vi "Browser_for_resources.vi"() -> ()   [LabVIEW 2015]
uses:
  Type Definitions/Data.ctl
  <vilib>/nisyscfg/Close (System).vi
  <vilib>/nisyscfg/nisyscfg.lvlib
panel:
  in  "Tab Control":enum32{"DAQmx", "SERIAL", "GPIB"}(tab)
  out "DAQ devices":bool caption="DAQ devices > 8"
  in  "List DAQ Rsrcs":bool
  out "ProdName":string[](array[string])
  out "DevName":string[](array[string])
  out "DAQ Mess":string caption="Messages"
  in  "Rename DAQ Rsrcs":bool
  in  "DevSerialNum":string
  out "Changed?":bool
  in  "New DevName":string
  out "DevSerialNum":string[](array[string])
  out "SER Mess":string caption="Messages"
  out "COM ports":string[](array[string])
  out "Serial I/F name":string[](array[string]) caption="Interface Instrument Name (RS232)"
  out "Serial Inst ID":string[](array[string]) caption="Instrument ID (RS232)"
  out "Serial List":string[](array[string]) caption="VISA Resource Name (RS232)"
  in  "List SERIAL Rsrcs":bool
  out "SERports >12":bool caption="SERIAL ports > 8"
  out "VISA List":string[](array[string]) caption="VISA Resources list"
  out "GPIB ports >12":bool caption="GPIB ports >8"
  out "Pr. Address":u16[](array[numeric])
  out "GPIB Inst ID":string[](array[string]) caption="Instrument ID (GPIB)"
  out "GPIB I/F name":string[](array[string]) caption="Interface Instrument Name (GPIB)"
  out "GPIB List":string[](array[string]) caption="VISA Resource Name (GPIB)"
  in  "List GPIB Rsrcs":bool
  out "GPIB Mess":string caption="Messages"
  out "VISA List 2":string[](array[string]) caption="VISA Resources list"
  in  "Exit":bool
  # "Browser for Resources (DAQmx, GPIB (INSTR) & SERIAL(INSTR)"
  # "Change DevName"
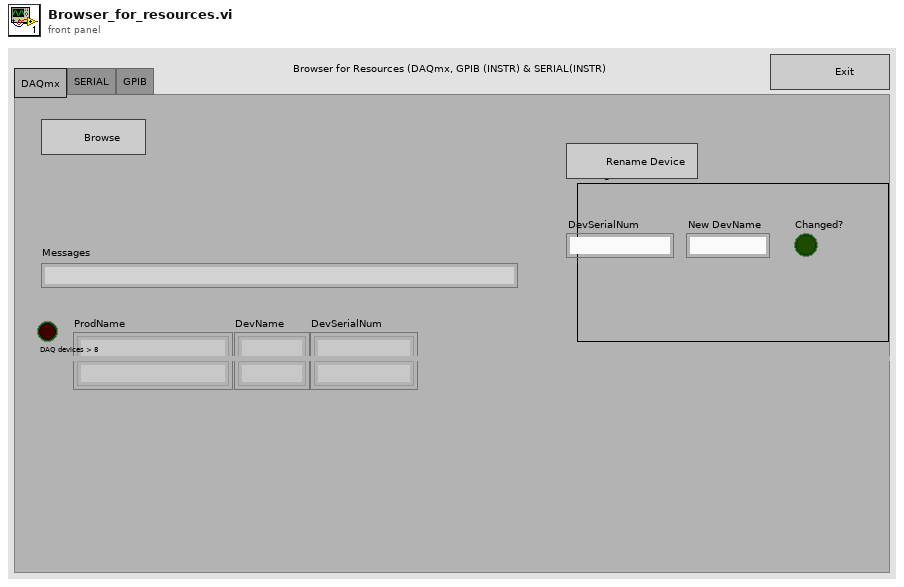
[diagram p1: front panel]
types:
  T1 = typedef "Data.ctl" = cluster{"Resources out":refnum<k20>[], "ProdName":string[], "DAQ Session":refnum<k21>, "DevName":string[], "DAQ Mess":string, "Changed?":bool, "VISA Rsrc":string[], "SERIAL Rsrc":string[], "SERIAL Inst ID":string[], "COM ports":string[], "SERIAL I/F name":string[], "SERIAL rows":u32, "SERIAL Mess":string, "GPIB Rsrc":string[], "GPIB Inst ID":string[], "Pr. Address":u16[], "GPIB I/F name":string[], "GPIB Mess":string, "GPIB rows":u32, "SerialNum":string[]}
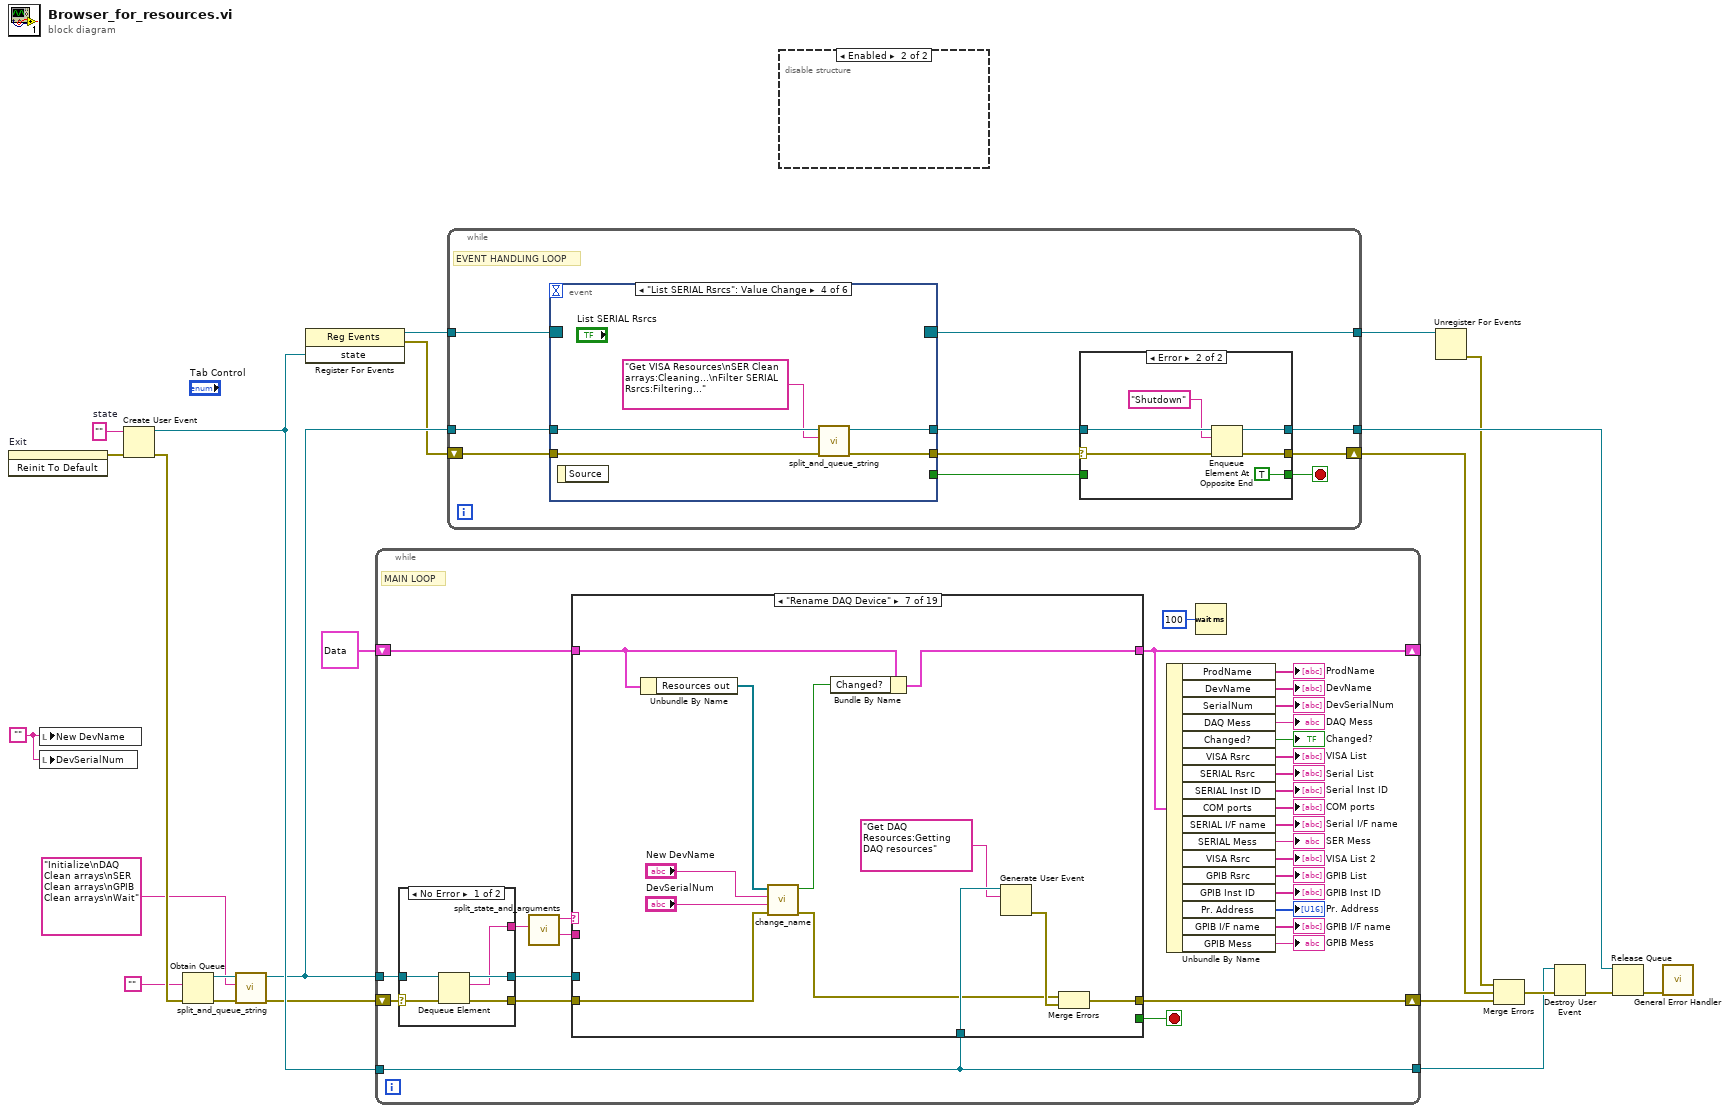
[diagram p0: block diagram]
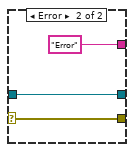
[diagram p3: hidden frame]
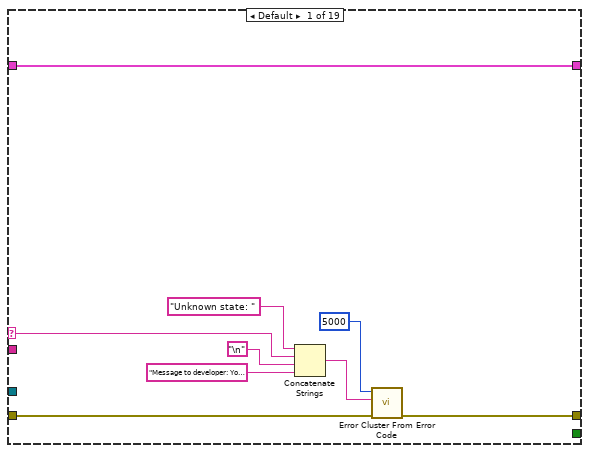
[diagram p4: hidden frame]
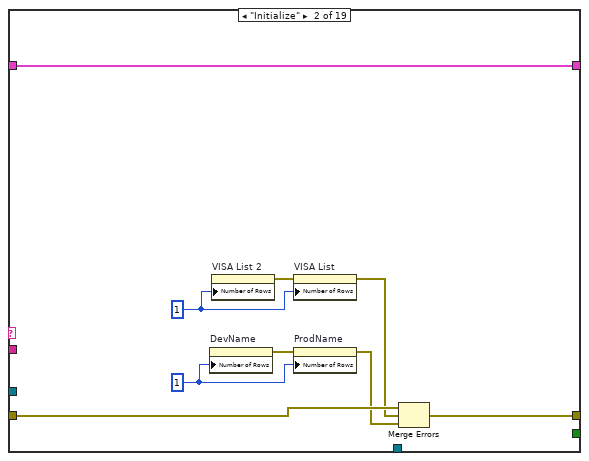
[diagram p5: hidden frame]
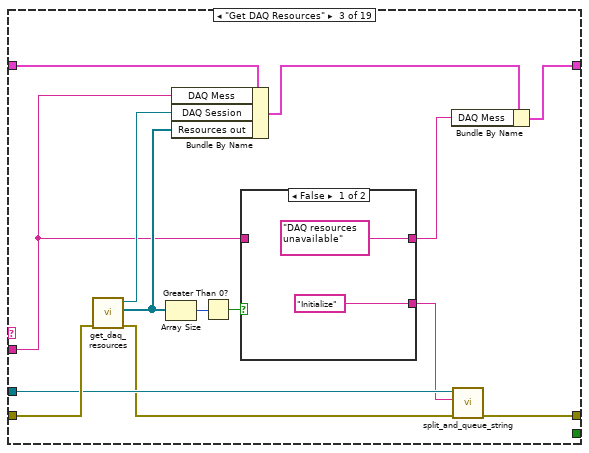
[diagram p6: hidden frame]
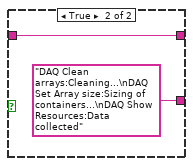
[diagram p7: hidden frame]
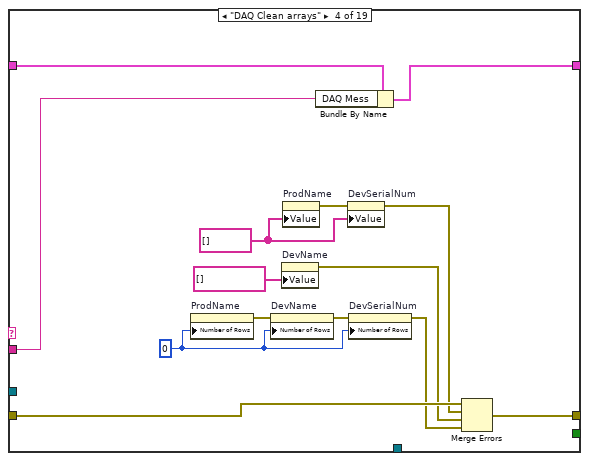
[diagram p8: hidden frame]
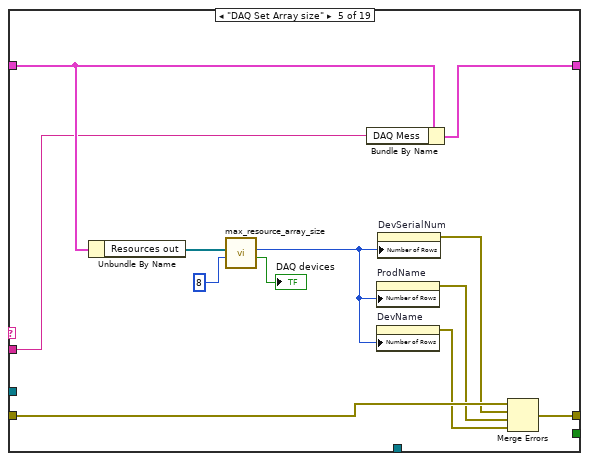
[diagram p9: hidden frame]
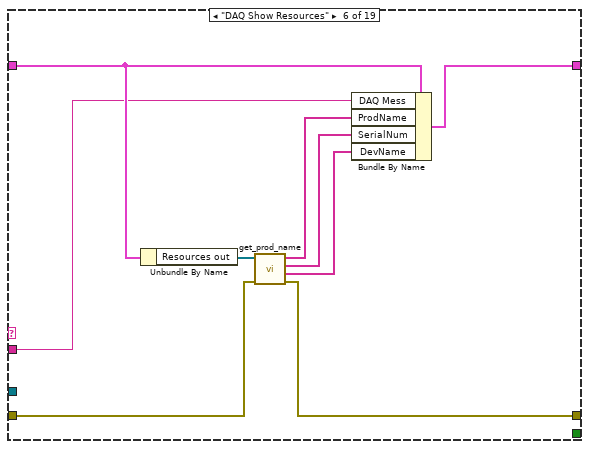
[diagram p10: hidden frame]
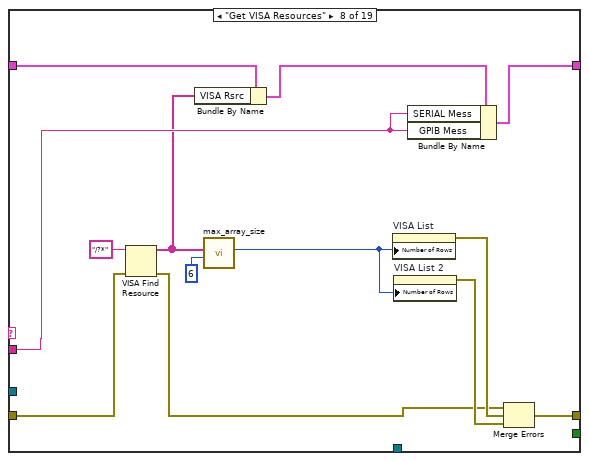
[diagram p11: hidden frame]
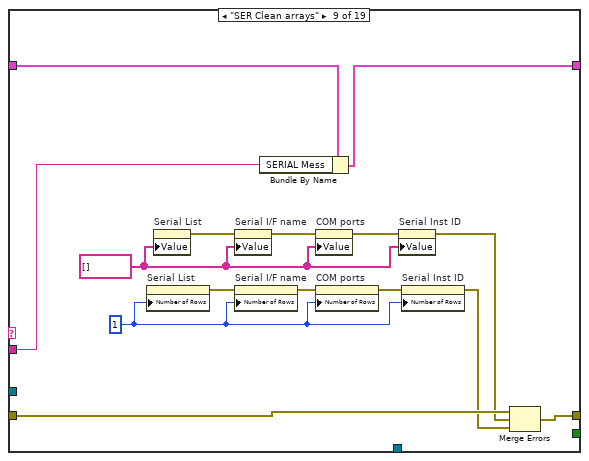
[diagram p12: hidden frame]
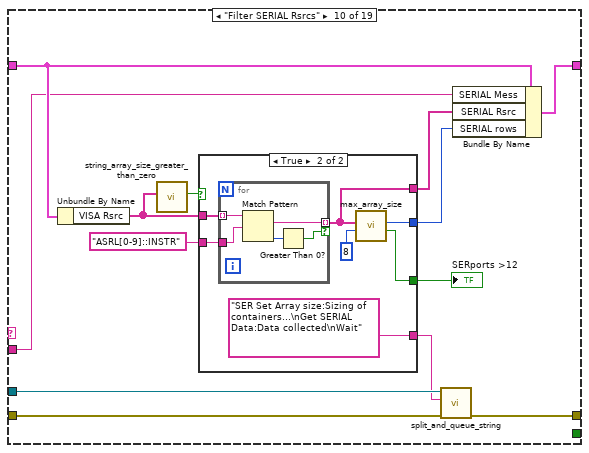
[diagram p13: hidden frame]
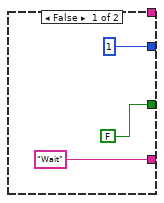
[diagram p14: hidden frame]
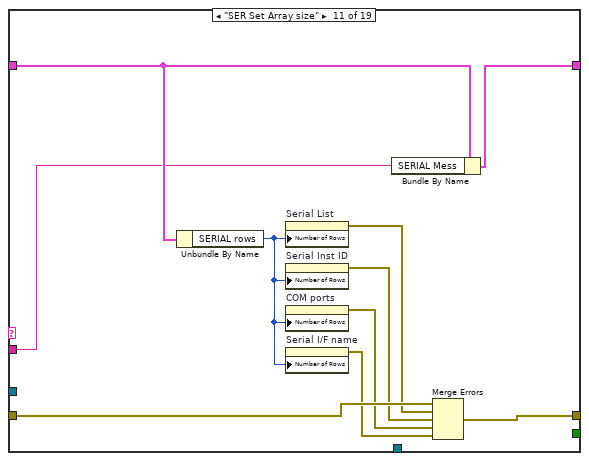
[diagram p15: hidden frame]
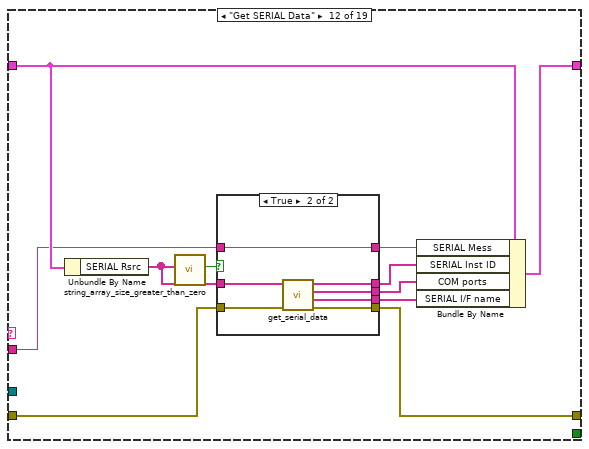
[diagram p16: hidden frame]
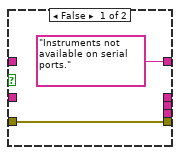
[diagram p17: hidden frame]
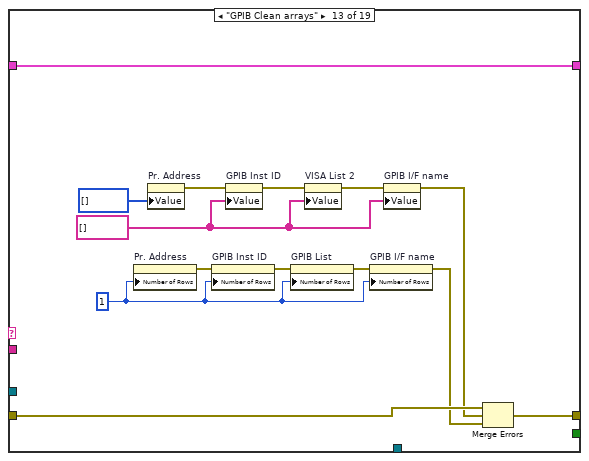
[diagram p18: hidden frame]
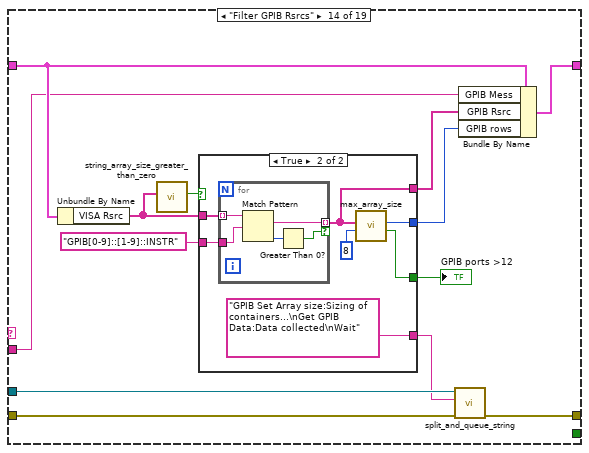
[diagram p19: hidden frame]
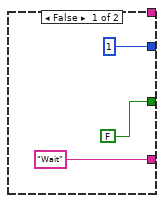
[diagram p20: hidden frame]
diagram:
  w1 = ""
  w13 = ""  # state
  n1 = invoke on="Exit" class="Bool (strict)" method="Reinit To Default"() -> (error out=w4:errorcluster)  [unwired: 3 in, 2 out]
  n2 = local write "New DevName"(w1) -> ()
  n3 = local write "DevSerialNum"(w1) -> ()
  n4 = Create User Event(user event datatype=w13, error in=w4) -> (user event=w23:refnum<user-event>, error out=w5:errorcluster)
  n5 = Obtain Queue(element data type="", error in (no error)=w5) -> (queue out=w21:refnum<queue>, error out=w22:errorcluster)  [unwired: 3 in, 1 out]
  n6 = call "split_and_queue_string.vi"("error in (no error)"=w22, "program string"="Initialize\nDAQ Clean arrays\nSER Clean arrays\nGPIB Clean arrays\nWait", "queue in"=w21) -> ("error out"=w6:errorcluster, "queue out"=w16:refnum<queue>)  [unwired: 7 in]
  n7 = register-events(w23) -> (reference out=w14:refnum<event-registration>, error out=w7:errorcluster)  [unwired: 2 in]
  n8 = while {
    shift-right: [w51] -> w20
    shift-left: w6 -> [w53]
    tunnel: w16 -> [w49]
    shift-right: [w43] -> _
    shift-left: T1 {"Resources out"=[], "ProdName"=[], "DAQ Session"="", "DevName"=[], "DAQ Mess"="", "Changed?"=FALSE, "VISA Rsrc"=[], "SERIAL Rsrc"=[], "SERIAL Inst ID"=[], "COM ports"=[], "SERIAL I/F name"=[], "SERIAL rows"=0, "SERIAL Mess"="", "GPIB Rsrc"=[], "GPIB Inst ID"=[], "Pr. Address"=[], "GPIB I/F name"=[], "GPIB Mess"="", "GPIB rows"=0, "SerialNum"=[]} -> [w44]
    tunnel: w23 -> [w24]
    tunnel: [w24] -> w8
    stop <- w50 stop-if-true
    # "MAIN LOOP"
    n9 = case shown="No Error" w53 {
      selector: w53 -> [w58 w61]
      tunnel: [w55 w61] -> w52
      tunnel: w49 -> [w57 w59]
      tunnel: [w54 "Error"] -> w47
      tunnel: [w56 w59] -> w48
      frame No Error {
        n10 = Dequeue Element(queue=w57, error in (no error)=w58) -> (queue out=w56:refnum<queue>, element=w54:string, error out=w55:errorcluster)  [unwired: 1 in, 1 out]
      }
      frame Error {
      }
    }
    n11 = call "split_state_and_arguments.vi"("String"=w47) -> ("Arguments"=w45:string, "State"=w46:string)  [unwired: 9 in]
    n12 = case shown="\"Rename DAQ Device\"" w46 {
      selector: w46 -> [w62 _ _ _ _ _ _ _ _ _ _ _ _ _ _ _ _ _ _]
      tunnel: w52 -> [w65 w79 w91 w111 w123 w125 w143 w155 w170 w177 w210 w218 w244 w250 w282 w290 w304 w306 w334]
      tunnel: [w64 w78 w88 w107 w122 w124 w137 w154 w169 w173 w209 w217 w236 w246 w281 w289 w304 w310 w335] -> w51
      tunnel: [_ _ _ _ _ _ _ _ _ _ _ _ _ _ _ _ _ _ w333] -> w50
      tunnel: w48 -> [_ _ w86 _ _ _ _ _ _ w176 _ _ _ w249 _ _ _ w314 _]
      tunnel: w45 -> [_ _ w80 w98 w117 w129 _ w148 w160 w175 w201 w212 _ w248 w273 w284 _ _ w327]
      tunnel: w44 -> [w70 w71 w93 w100 w121 w131 w140 w156 w162 w181 w203 w216 w243 w254 w275 w288 w303 w313 w332]
      tunnel: [w70 w71 w82 w99 w120 w130 w139 w150 w161 w180 w202 w215 w243 w253 w274 w287 w303 w312 w331] -> w43
      tunnel: w24 -> [_ _ _ _ _ _ w135 _ _ _ _ _ _ _ _ _ _ _ _]
      frame Default {
        n13 = Concatenate Strings("Unknown state: " ("string"), w62, "\n", "Message to developer: You typed a state name that is not recognized.") -> (w68:string)
        n14 = call <vilib>:"Error Cluster From Error Code.vi"("error in (no error)"=w65, "error message (\"\")"=w68, "error code (0)"=5000) -> ("error out"=w64:errorcluster)  [unwired: 6 in]
      }
      frame "Initialize" {
        w75 = u32 1 ("Number of Rows")
        w77 = u32 1 ("Number of Rows")
        n15 = property on="DevName" class="Arr (strict)"("Number of Rows"=w77) -> (error out=w73:errorcluster)  [unwired: 2 in, 1 out]
        n16 = property on="VISA List 2" class="Arr (strict)"("Number of Rows"=w75) -> (error out=w76:errorcluster)  [unwired: 2 in, 1 out]
        n17 = property on="VISA List" class="Arr (strict)"(error in=w76, "Number of Rows"=w75) -> (error out=w74:errorcluster)  [unwired: 1 in, 1 out]
        n18 = property on="ProdName" class="Arr (strict)"(error in=w73, "Number of Rows"=w77) -> (error out=w72:errorcluster)  [unwired: 1 in, 1 out]
        n19 = Merge Errors(w79, w74, w72) -> (w78:errorcluster)
      }
      frame "Get DAQ Resources" {
        n20 = call "get_daq_resources.vi"("error in (no error)"=w91) -> ("error out"=w85:errorcluster, "Resources out"=w90:refnum<k20>[], "Refnum out"=w92:refnum<k21>)  [unwired: 8 in]
        n21 = Array Size(array=w90) -> (size(s)=w89:i32)
        n22 = Bundle By Name(cluster=w93, "DAQ Mess"=w80, "DAQ Session"=w92, "Resources out"=w90) -> (w83:T1)
        n23 = Greater Than 0?(x=w89) -> (x > 0?=w87:bool)
        n24 = case shown="False" w87 {
          tunnel: ["Initialize" "DAQ Clean arrays:Cleaning...\nDAQ Set Array size:Sizing of containers...\nDAQ Show Resources:Data collected"] -> w84
          tunnel: ["DAQ resources unavailable" w96] -> w81
          tunnel: w80 -> [_ w96]
          frame False {
          }
          frame True {
          }
        }
        n25 = Bundle By Name(cluster=w83, "DAQ Mess"=w81) -> (w82:T1)
        n26 = call "split_and_queue_string.vi"("error in (no error)"=w85, "program string"=w84, "queue in"=w86) -> ("error out"=w88:errorcluster)  [unwired: 7 in, 1 out]
      }
      frame "DAQ Clean arrays" {
        w101 = u32 0 ("Number of Rows")
        w109 = string[] []
        n27 = property on="ProdName" class="Arr (strict)"("Number of Rows"=w101) -> (error out=w102:errorcluster)  [unwired: 2 in, 1 out]
        n28 = property on="DevName" class="Arr (strict)"(error in=w102, "Number of Rows"=w101) -> (error out=w104:errorcluster)  [unwired: 1 in, 1 out]
        n29 = property on="DevName" class="Arr (strict)"("Value"=tag[] []) -> (error out=w105:errorcluster)  [unwired: 2 in, 1 out]
        n30 = property on="ProdName" class="Arr (strict)"("Value"=w109) -> (error out=w110:errorcluster)  [unwired: 2 in, 1 out]
        n31 = Bundle By Name(cluster=w100, "DAQ Mess"=w98) -> (w99:T1)
        n32 = property on="DevSerialNum" class="Arr (strict)"(error in=w110, "Value"=w109) -> (error out=w106:errorcluster)  [unwired: 1 in, 1 out]
        n33 = property on="DevSerialNum" class="Arr (strict)"(error in=w104, "Number of Rows"=w101) -> (error out=w103:errorcluster)  [unwired: 1 in, 1 out]
        n34 = Merge Errors(w111, w106, w105, w103) -> (w107:errorcluster)
      }
      frame "DAQ Set Array size" {
        n35 = Unbundle By Name(w121) -> ("Resources out"=w113:refnum<k20>[])
        n36 = call "max_resource_array_size.vi"("max rows"=u32 8, "Resources in"=w113) -> ("size > max rows"=→"DAQ devices":bool, "array size"=w112:u32)  [unwired: 8 in]
        n37 = Bundle By Name(cluster=w121, "DAQ Mess"=w117) -> (w120:T1)
        n38 = property on="ProdName" class="Arr (strict)"("Number of Rows"=w112) -> (error out=w119:errorcluster)  [unwired: 2 in, 1 out]
        n39 = property on="DevName" class="Arr (strict)"("Number of Rows"=w112) -> (error out=w118:errorcluster)  [unwired: 2 in, 1 out]
        n40 = property on="DevSerialNum" class="Arr (strict)"("Number of Rows"=w112) -> (error out=w116:errorcluster)  [unwired: 2 in, 1 out]
        n41 = Merge Errors(w123, w116, w119, w118) -> (w122:errorcluster)
      }
      frame "DAQ Show Resources" {
        n42 = Unbundle By Name(w131) -> ("Resources out"=w132:refnum<k20>[])
        n43 = call "get_prod_name.vi"("error in (no error)"=w125, "Resources in"=w132) -> ("error out"=w124:errorcluster, "Alias"=w126:string[], "SerialNum"=w127:string[], "ProdName"=w128:string[])  [unwired: 6 in]
        n44 = Bundle By Name(cluster=w131, "DAQ Mess"=w129, "ProdName"=w128, "SerialNum"=w127, "DevName"=w126) -> (w130:T1)
      }
      frame "Rename DAQ Device" {
        n45 = Unbundle By Name(w140) -> ("Resources out"=w144:refnum<k20>[])
        n46 = call "change_name.vi"("error in (no error)"=w143, "SerialNum"="DevSerialNum", "New Dev Name"="New DevName", "Resources in"=w144) -> ("error out"=w133:errorcluster, "Changed?"=w138:bool)  [unwired: 6 in]
        n47 = Bundle By Name(cluster=w140, "Changed?"=w138) -> (w139:T1)
        n48 = Generate User Event(user event=w135, event data cluster="Get DAQ Resources:Getting DAQ resources" ("element")) -> (error out=w136:errorcluster)  [unwired: 2 in, 1 out]
        n49 = Merge Errors(w133, w136) -> (w137:errorcluster)
      }
      frame "Get VISA Resources" {
        n50 = VISA Find Resource(8:w155, 11:"/?*") -> (0:w149:errorcluster, 3:w147:string[])  [unwired: 1 in, 1 out]
        n51 = Bundle By Name(cluster=w156, "VISA Rsrc"=w147) -> (w151:T1)
        n52 = call "max_array_size.vi"("max rows"=u32 6 ("y"), "Array"=w147) -> ("array size"=w146:u32)  [unwired: 8 in, 1 out]
        n53 = property on="VISA List" class="Arr (strict)"("Number of Rows"=w146) -> (error out=w153:errorcluster)  [unwired: 2 in, 1 out]
        n54 = property on="VISA List 2" class="Arr (strict)"("Number of Rows"=w146) -> (error out=w152:errorcluster)  [unwired: 2 in, 1 out]
        n55 = Bundle By Name(cluster=w151, "SERIAL Mess"=w148, "GPIB Mess"=w148) -> (w150:T1)
        n56 = Merge Errors(w149, w153, w152) -> (w154:errorcluster)
      }
      frame "SER Clean arrays" {
        w165 = string[] []
        w158 = u32 1
        n57 = property on="Serial List" class="Arr (strict)"("Number of Rows"=w158) -> (error out=w159:errorcluster)  [unwired: 2 in, 1 out]
        n58 = property on="Serial List" class="Arr (strict)"("Value"=w165) -> (error out=w166:errorcluster)  [unwired: 2 in, 1 out]
        n59 = property on="Serial I/F name" class="Arr (strict)"(error in=w166, "Value"=w165) -> (error out=w167:errorcluster)  [unwired: 1 in, 1 out]
        n60 = property on="Serial I/F name" class="Arr (strict)"(error in=w159, "Number of Rows"=w158) -> (error out=w172:errorcluster)  [unwired: 1 in, 1 out]
        n61 = Bundle By Name(cluster=w162, "SERIAL Mess"=w160) -> (w161:T1)
        n62 = property on="COM ports" class="Arr (strict)"(error in=w167, "Value"=w165) -> (error out=w164:errorcluster)  [unwired: 1 in, 1 out]
        n63 = property on="COM ports" class="Arr (strict)"(error in=w172, "Number of Rows"=w158) -> (error out=w171:errorcluster)  [unwired: 1 in, 1 out]
        n64 = property on="Serial Inst ID" class="Arr (strict)"(error in=w164, "Value"=w165) -> (error out=w163:errorcluster)  [unwired: 1 in, 1 out]
        n65 = property on="Serial Inst ID" class="Arr (strict)"(error in=w171, "Number of Rows"=w158) -> (error out=w168:errorcluster)  [unwired: 1 in, 1 out]
        n66 = Merge Errors(w170, w163, w168) -> (w169:errorcluster)
      }
      frame "Filter SERIAL Rsrcs" {
        n67 = Unbundle By Name(w181) -> ("VISA Rsrc"=w178:string[])
        n68 = call "string_array_size_greater_than_zero.vi"("array"=w178) -> ("size > 0?"=w179:bool)  [unwired: 10 in]
        n69 = case shown="True" w179 {
          tunnel: [FALSE ("size > max rows") w195] -> w185
          tunnel: [u32 1 ("array size") w194] -> w184
          tunnel: [_ w193] -> w183
          tunnel: "ASRL[0-9]::INSTR" ("regular expression") -> [_ w192]
          tunnel: w178 -> [_ w191]
          tunnel: ["Wait" "SER Set Array size:Sizing of containers...\nGet SERIAL Data:Data collected\nWait"] -> w174
          frame False {
          }
          frame True {
            n70 = for {
              tunnel: [w200] -> w193 mode=indexing if=w198
              tunnel: w191 -> [w197] mode=indexing
              tunnel: w192 -> [w196]
              n71 = Match Pattern(string=w197, regular expression=w196) -> (match substring=w200:string, offset past match=w199:i32)  [unwired: 1 in, 2 out]
              n72 = Greater Than 0?(x=w199) -> (x > 0?=w198:bool)
            }
            n73 = call "max_array_size.vi"("max rows"=u32 8, "Array"=w193) -> ("size > max rows"=w195:bool, "array size"=w194:u32)  [unwired: 8 in]
          }
        }
        "SERports >12" <- w185
        n74 = call "split_and_queue_string.vi"("error in (no error)"=w177, "program string"=w174, "queue in"=w176) -> ("error out"=w173:errorcluster)  [unwired: 7 in, 1 out]
        n75 = Bundle By Name(cluster=w181, "SERIAL Mess"=w175, "SERIAL Rsrc"=w183, "SERIAL rows"=w184) -> (w180:T1)
      }
      frame "SER Set Array size" {
        n76 = Unbundle By Name(w203) -> ("SERIAL rows"=w205:u32)
        n77 = property on="Serial List" class="Arr (strict)"("Number of Rows"=w205) -> (error out=w204:errorcluster)  [unwired: 2 in, 1 out]
        n78 = property on="Serial Inst ID" class="Arr (strict)"("Number of Rows"=w205) -> (error out=w206:errorcluster)  [unwired: 2 in, 1 out]
        n79 = property on="COM ports" class="Arr (strict)"("Number of Rows"=w205) -> (error out=w207:errorcluster)  [unwired: 2 in, 1 out]
        n80 = property on="Serial I/F name" class="Arr (strict)"("Number of Rows"=w205) -> (error out=w208:errorcluster)  [unwired: 2 in, 1 out]
        n81 = Bundle By Name(cluster=w203, "SERIAL Mess"=w201) -> (w202:T1)
        n82 = Merge Errors(w210, w204, w206, w207, w208) -> (w209:errorcluster)
      }
      frame "Get SERIAL Data" {
        n83 = Unbundle By Name(w216) -> ("SERIAL Rsrc"=w213:string[])
        n84 = call "string_array_size_greater_than_zero.vi"("array"=w213) -> ("size > 0?"=w214:bool)  [unwired: 10 in]
        n85 = case shown="True" w214 {
          tunnel: w218 -> [w223 w230]
          tunnel: [w223 w229] -> w217
          tunnel: w213 -> [_ w228]
          tunnel: [_ w227] -> w219
          tunnel: ["Instruments not available on serial ports." w226] -> w211
          tunnel: w212 -> [_ w226]
          tunnel: [_ w225] -> w220
          tunnel: [_ w224] -> w221
          frame False {
          }
          frame True {
            n86 = call "get_serial_data.vi"("error in (no error)"=w230, "SERIAL Rsrc"=w228) -> ("error out"=w229:errorcluster, "I/F name"=w225:string[], "COM ports"=w224:string[], "Inst ID"=w227:string[])  [unwired: 6 in]
          }
        }
        n87 = Bundle By Name(cluster=w216, "SERIAL Mess"=w211, "SERIAL Inst ID"=w219, "COM ports"=w221, "SERIAL I/F name"=w220) -> (w215:T1)
      }
      frame "GPIB Clean arrays" {
        w231 = u32 1
        w238 = string[] [] ("GPIB Inst ID")
        n88 = property on="Pr. Address" class="Arr (strict)"("Number of Rows"=w231) -> (error out=w237:errorcluster)  [unwired: 2 in, 1 out]
        n89 = property on="Pr. Address" class="Arr (strict)"("Value"=u16[] [] ("Pr. Address")) -> (error out=w241:errorcluster)  [unwired: 2 in, 1 out]
        n90 = property on="GPIB Inst ID" class="Arr (strict)"(error in=w237, "Number of Rows"=w231) -> (error out=w233:errorcluster)  [unwired: 1 in, 1 out]
        n91 = property on="GPIB Inst ID" class="Arr (strict)"(error in=w241, "Value"=w238) -> (error out=w240:errorcluster)  [unwired: 1 in, 1 out]
        n92 = property on="GPIB List" class="Arr (strict)"(error in=w233, "Number of Rows"=w231) -> (error out=w232:errorcluster)  [unwired: 1 in, 1 out]
        n93 = property on="VISA List 2" class="Arr (strict)"(error in=w240, "Value"=w238) -> (error out=w239:errorcluster)  [unwired: 1 in, 1 out]
        n94 = property on="GPIB I/F name" class="Arr (strict)"(error in=w232, "Number of Rows"=w231) -> (error out=w235:errorcluster)  [unwired: 1 in, 1 out]
        n95 = property on="GPIB I/F name" class="Arr (strict)"(error in=w239, "Value"=w238) -> (error out=w234:errorcluster)  [unwired: 1 in, 1 out]
        n96 = Merge Errors(w244, w234, w235) -> (w236:errorcluster)
      }
      frame "Filter GPIB Rsrcs" {
        n97 = Unbundle By Name(w254) -> ("VISA Rsrc"=w251:string[])
        n98 = call "string_array_size_greater_than_zero.vi"("array"=w251) -> ("size > 0?"=w252:bool)  [unwired: 10 in]
        n99 = case shown="True" w252 {
          tunnel: [FALSE ("size > max rows") w267] -> w245
          tunnel: [u32 1 ("array size") w266] -> w257
          tunnel: [_ w265] -> w256
          tunnel: "GPIB[0-9]::[1-9]::INSTR" ("regular expression") -> [_ w264]
          tunnel: w251 -> [_ w263]
          tunnel: ["Wait" "GPIB Set Array size:Sizing of containers...\nGet GPIB Data:Data collected\nWait"] -> w247
          frame False {
          }
          frame True {
            n100 = for {
              tunnel: [w272] -> w265 mode=indexing if=w270
              tunnel: w263 -> [w269] mode=indexing
              tunnel: w264 -> [w268]
              n101 = Match Pattern(string=w269, regular expression=w268) -> (match substring=w272:string, offset past match=w271:i32)  [unwired: 1 in, 2 out]
              n102 = Greater Than 0?(x=w271) -> (x > 0?=w270:bool)
            }
            n103 = call "max_array_size.vi"("max rows"=u32 8, "Array"=w265) -> ("size > max rows"=w267:bool, "array size"=w266:u32)  [unwired: 8 in]
          }
        }
        "GPIB ports >12" <- w245
        n104 = call "split_and_queue_string.vi"("error in (no error)"=w250, "program string"=w247, "queue in"=w249) -> ("error out"=w246:errorcluster)  [unwired: 7 in, 1 out]
        n105 = Bundle By Name(cluster=w254, "GPIB Mess"=w248, "GPIB Rsrc"=w256, "GPIB rows"=w257) -> (w253:T1)
      }
      frame "GPIB Set Array size" {
        n106 = Unbundle By Name(w275) -> ("GPIB rows"=w277:u32)
        n107 = property on="GPIB List" class="Arr (strict)"("Number of Rows"=w277) -> (error out=w276:errorcluster)  [unwired: 2 in, 1 out]
        n108 = property on="GPIB Inst ID" class="Arr (strict)"("Number of Rows"=w277) -> (error out=w278:errorcluster)  [unwired: 2 in, 1 out]
        n109 = property on="Pr. Address" class="Arr (strict)"("Number of Rows"=w277) -> (error out=w279:errorcluster)  [unwired: 2 in, 1 out]
        n110 = property on="GPIB I/F name" class="Arr (strict)"("Number of Rows"=w277) -> (error out=w280:errorcluster)  [unwired: 2 in, 1 out]
        n111 = Bundle By Name(cluster=w275, "GPIB Mess"=w273) -> (w274:T1)
        n112 = Merge Errors(w282, w276, w278, w279, w280) -> (w281:errorcluster)
      }
      frame "Get GPIB Data" {
        n113 = Unbundle By Name(w288) -> ("GPIB Rsrc"=w285:string[])
        n114 = call "string_array_size_greater_than_zero.vi"("array"=w285) -> ("size > 0?"=w286:bool)  [unwired: 10 in]
        n115 = case shown="True" w286 {
          tunnel: w290 -> [w295 w302]
          tunnel: [w295 w301] -> w289
          tunnel: w285 -> [_ w300]
          tunnel: [_ w299] -> w291
          tunnel: ["Instruments not available on gpib ports." w298] -> w283
          tunnel: w284 -> [_ w298]
          tunnel: [_ w297] -> w292
          tunnel: [_ w296] -> w293
          frame False {
          }
          frame True {
            n116 = call "get_gpib_data.vi"("error in (no error)"=w302, "GPIB Rsrc"=w300) -> ("error out"=w301:errorcluster, "GPIB I/F name"=w297:string[], "Primary Address"=w296:u16[], "GPIB Inst ID"=w299:string[])  [unwired: 6 in]
          }
        }
        n117 = Bundle By Name(cluster=w288, "GPIB Mess"=w283, "GPIB Inst ID"=w291, "Pr. Address"=w293, "GPIB I/F name"=w292) -> (w287:T1)
      }
      frame "Wait" {
      }
      frame "Error" {
        n118 = case shown="No Error" w306 {
          selector: w306 -> [w315 w318]
          tunnel: ["" w322] -> w311
          tunnel: ["Wait" w321] -> w305
          tunnel: [w315 w320] -> w309
          frame No Error {
          }
          frame Error {
            n119 = Unbundle By Name(w318) -> ("code"=w319:i32)
            n120 = case shown="-1073807343" w319 {
              tunnel: ["" "It is possible that there are no instruments connected or they are switched off."] -> w322
              tunnel: ["Wait" "Wait"] -> w321
              frame Default {
              }
              frame -1073807343 {
              }
            }
            n121 = call <vilib>:"Clear Errors.vi"("error in (no error)"=w318, "specific error code to clear (0: all)"=w319) -> ("error out"=w320:errorcluster)  [unwired: 4 in, 1 out]
          }
        }
        n122 = Bundle By Name(cluster=w313, "SERIAL Mess"=w311, "GPIB Mess"=w311) -> (w312:T1)
        n123 = Flush Queue(queue=w314, error in (no error)=w309) -> (queue out=w308:refnum<queue>, error out=w307:errorcluster)  [unwired: 1 out]
        n124 = call "split_and_queue_string.vi"("error in (no error)"=w307, "program string"=w305, "queue in"=w308) -> ("error out"=w310:errorcluster)  [unwired: 7 in, 1 out]
      }
      frame "Shutdown" {
        w333 = TRUE
        n125 = Bundle By Name(cluster=w332, "DAQ Mess"=w327, "SERIAL Mess"=w327, "GPIB Mess"=w327) -> (w331:T1)
        n126 = Unbundle By Name(w331) -> ("DAQ Session"=w330:refnum<k21>)
        n127 = property on="Exit" class="Bool (strict)"("Val(Sgnl)"=w333) -> (error out=w328:errorcluster)  [unwired: 2 in, 1 out]
        n128 = call-poly <vilib>:"Close.vi"("Session in"=w330) -> ("error out"=w329:errorcluster)  [unwired: 10 in]
        n129 = Merge Errors(w334, w329, w328) -> (w335:errorcluster)
      }
    }
    n130 = Unbundle By Name(w43) -> ("ProdName"=→"ProdName":string[], "DevName"=→"DevName":string[], "SerialNum"=→"DevSerialNum":string[], "DAQ Mess"=→"DAQ Mess":string, "Changed?"=→"Changed?":bool, "VISA Rsrc"=→"VISA List":string[], "SERIAL Rsrc"=→"Serial List":string[], "SERIAL Inst ID"=→"Serial Inst ID":string[], "COM ports"=→"COM ports":string[], "SERIAL I/F name"=→"Serial I/F name":string[], "SERIAL Mess"=→"SER Mess":string, "VISA Rsrc"=→"VISA List 2":string[], "GPIB Rsrc"=→"GPIB List":string[], "GPIB Inst ID"=→"GPIB Inst ID":string[], "Pr. Address"=→"Pr. Address":u16[], "GPIB I/F name"=→"GPIB I/F name":string[], "GPIB Mess"=→"GPIB Mess":string)
    n131 = Wait (ms)(milliseconds to wait=u32 100) -> ()  [unwired: 1 out]
  }
  n132 = while {
    shift-right: [w343] -> w19
    shift-left: w7 -> [w345]
    tunnel: w16 -> [w340]
    tunnel: [w338] -> w18
    tunnel: w14 -> [w337]
    tunnel: [w336] -> w12
    stop <- w342 stop-if-true
    # "EVENT HANDLING LOOP"
    n133 = event shown="[3] \"List SERIAL Rsrcs\": Value Change" {
      selector: w337 -> [_ _ _ _ _ _]
      dyn-events: [_ _ _ _ _ _] -> w336
      timeout: _ -> [_ _ _ _ _ _]
      tunnel: w345 -> [w357 w365 w370 w373 w378 w387]
      tunnel: [w360 w363 w368 w376 w381 w386] -> w344
      tunnel: [_ _ _ _ _ TRUE] -> w341
      tunnel: w340 -> [w359 w366 w371 w374 w379 w385]
      tunnel: [w361 w364 w369 w375 w380 w384] -> w339
      event "List DAQ Rsrcs": Value Change {
        n134 = event-data() -> ()  [unwired: 1 in, 1 out]
        n135 = Flush Queue(queue=w359, error in (no error)=w357) -> (queue out=w358:refnum<queue>, error out=w356:errorcluster)  [unwired: 1 out]
        n136 = call "split_and_queue_string.vi"("error in (no error)"=w356, "program string"="Get DAQ Resources:Getting DAQ resources" ("element"), "queue in"=w358) -> ("error out"=w360:errorcluster, "queue out"=w361:refnum<queue>)  [unwired: 7 in]
      }
      event User Event {
        n137 = event-data() -> ("state"=w362:string)  [unwired: 1 in]
        n138 = call "split_and_queue_string.vi"("error in (no error)"=w365, "program string"=w362, "queue in"=w366) -> ("error out"=w363:errorcluster, "queue out"=w364:refnum<queue>)  [unwired: 7 in]
      }
      event "Rename DAQ Rsrcs": Value Change {
        n139 = event-data() -> ()  [unwired: 1 in, 1 out]
        n140 = call "split_and_queue_string.vi"("error in (no error)"=w370, "program string"="Rename DAQ Device", "queue in"=w371) -> ("error out"=w368:errorcluster, "queue out"=w369:refnum<queue>)  [unwired: 7 in]
      }
      event "List SERIAL Rsrcs": Value Change {
        n141 = event-data() -> ()  [unwired: 1 in, 1 out]
        n142 = call "split_and_queue_string.vi"("error in (no error)"=w373, "program string"="Get VISA Resources\nSER Clean arrays:Cleaning...\nFilter SERIAL Rsrcs:Filtering...", "queue in"=w374) -> ("error out"=w376:errorcluster, "queue out"=w375:refnum<queue>)  [unwired: 7 in]
      }
      event "List GPIB Rsrcs": Value Change {
        n143 = event-data() -> ()  [unwired: 1 in, 1 out]
        n144 = call "split_and_queue_string.vi"("error in (no error)"=w378, "program string"="Get VISA Resources\nGPIB Clean arrays:Cleaning...\nFilter GPIB Rsrcs:Filtering...", "queue in"=w379) -> ("error out"=w381:errorcluster, "queue out"=w380:refnum<queue>)  [unwired: 7 in]
      }
      event "Exit": Value Change {
        n145 = event-data() -> ()  [unwired: 1 in, 1 out]
        n146 = Enqueue Element At Opposite End(queue=w385, element="Shutdown:Terminating...", error in (no error)=w387) -> (queue out=w384:refnum<queue>, error out=w386:errorcluster)  [unwired: 1 in, 1 out]
      }
    }
    n147 = case shown="Error" w344 {
      selector: w344 -> [w348 w354]
      tunnel: [w348 w353] -> w343
      tunnel: [w346 TRUE] -> w342
      tunnel: w341 -> [w346 _]
      tunnel: w339 -> [w347 w352]
      tunnel: [w347 w351] -> w338
      frame No Error {
      }
      frame Error {
        n148 = Enqueue Element At Opposite End(queue=w352, element="Shutdown", error in (no error)=w354) -> (queue out=w351:refnum<queue>, error out=w353:errorcluster)  [unwired: 1 in, 1 out]
      }
    }
  }
  n149 = disable-structure shown="Enabled" {
    frame Disabled {
    }
    frame Enabled {
    }
  }
  n150 = Unregister For Events(event registration refnum=w12) -> (error out=w11:errorcluster)  [unwired: 1 in]
  n151 = Merge Errors(w11, w19, w20) -> (w10:errorcluster)
  n152 = Destroy User Event(user event=w8, error in=w10) -> (error out=w9:errorcluster)
  n153 = Release Queue(queue=w18, error in (no error)=w9) -> (error out=w17:errorcluster)  [unwired: 1 in, 2 out]
  n154 = call <vilib>:"General Error Handler.vi"("error in (no error)"=w17) -> ()  [unwired: 10 in, 5 out]
